vi "Calibration_AH2700.vi"(4 "B-Feld":dbl=4.0, 5 "error in (no error)":errorcluster) -> (15 "Ausgabe-Cluster":T1={" I (A)"=-6.000000000000021, "Voltage"=0.143902, "B-Feld"=4.0, "Timestamp"=3443775799.1979947} {"Timestamp" format="%#_6f"}, 19 "error out":errorcluster)   [LabVIEW 2019]
uses:
  Instrument_Setup.vi
  Global/Global Variables/global.vi
  Instance           2 16Saved   Yokogawa .vi
  Global/Global Variables/Data_Display_global.vi
  <vilib>/Utility/file.llb/Write To Spreadsheet File (DBL).vi
panel:
  out "XY Graph":cluster{dbl[], dbl[]}(graph)={[-6.000000000000005, -4.990000000000027, -3.9901000000000244, -2.9900990000000083, -1.9999999999999865, -0.9900000000000079, 2.400857290751901e-15, 1.000000000000001, 2.0000000000000018, 3.0099999999999802, 4.009899999999982, 5.009900999999998, 6.00000000000002, 4.990000000000042, 3.9901000000000395, 2.999999999999979, 1.9900000000000007, 0.9999999999999987, -1.5439038936193583e-15, -1.0000000000000018, -2.0000000000000027, -3.009999999999981, -4.009899999999983, -5.009900999999999, -6.000000000000021], [0.1439003448275862, 0.14384071428571427, 0.14379167857142858, 0.14374593103448274, 0.14371203448275863, 0.14368321428571423, 0.1436658620689656, 0.1436561034482759, 0.14365485714285722, 0.14366034482758627, 0.14367178571428574, 0.1436978571428571, 0.14372814285714283, 0.14369535714285714, 0.1436752857142857, 0.14366071428571434, 0.14365396428571436, 0.14365448275862072, 0.14366448275862076, 0.14368586206896547, 0.1437107142857143, 0.14374785714285715, 0.14379375862068966, 0.1438423214285714, 0.1439047142857143]}
  in  "file path (dialog if empty)":path=path "D:/UserData/Matthias/Messungen/MgOZnO/130215/130215_259a_kalib4T_1.txt"
  out "Done":bool=TRUE
  out "Data":bool
  out "UI":dbl=-6.000000000000021
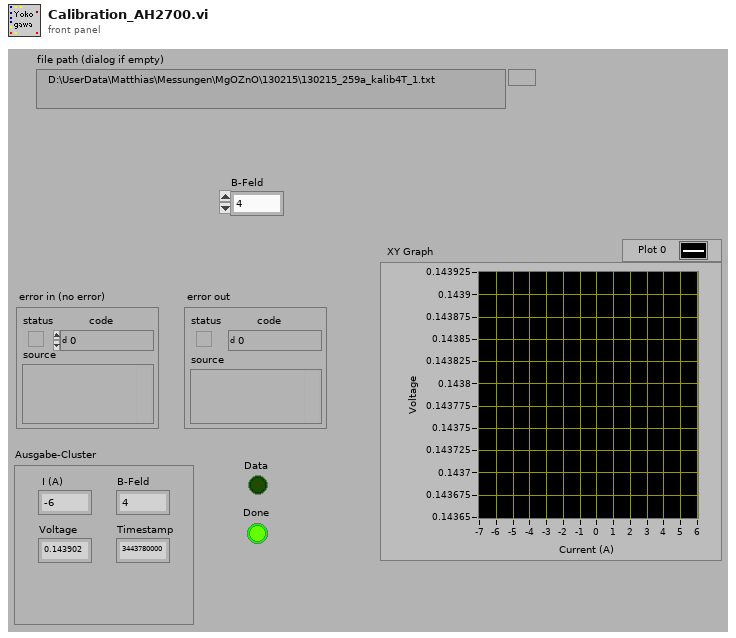
[diagram p1: front panel]
types:
  T1 = cluster{" I (A)":dbl, "Voltage":dbl, "B-Feld":dbl, "Timestamp":dbl}
  T2 = cluster{"UI":dbl, "Capacity":dbl, "B-Feld":dbl, dbl}
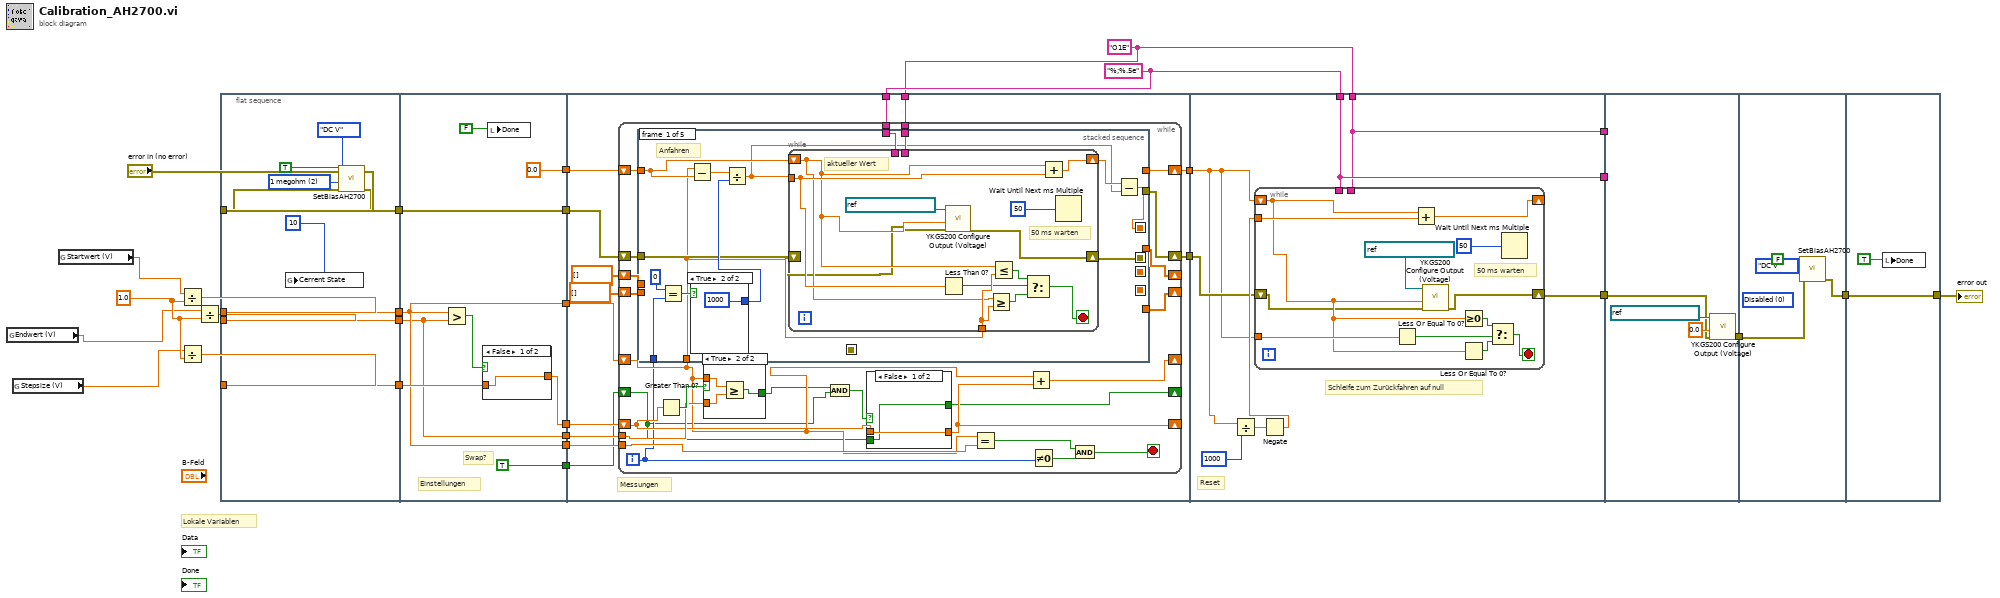
[diagram p0: block diagram]
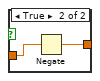
[diagram p2: hidden frame]
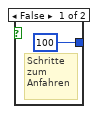
[diagram p3: hidden frame]
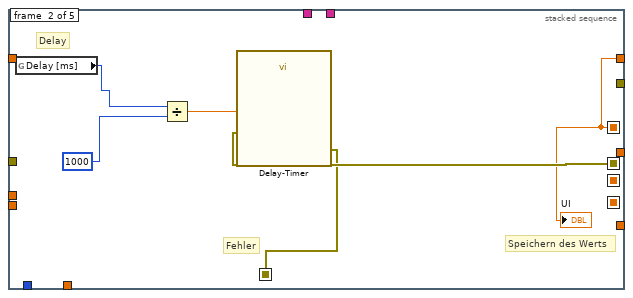
[diagram p4: hidden frame]
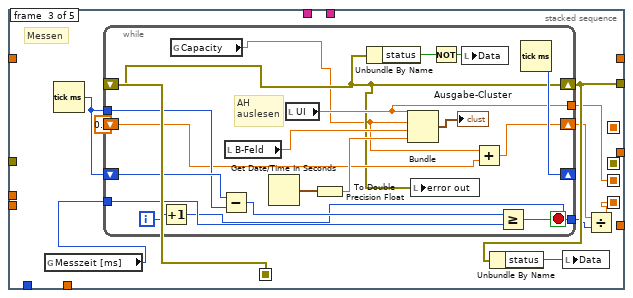
[diagram p5: hidden frame]
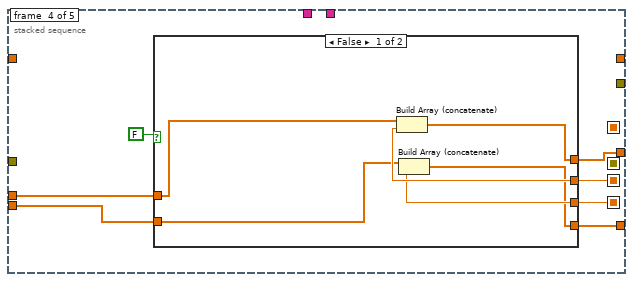
[diagram p6: hidden frame]
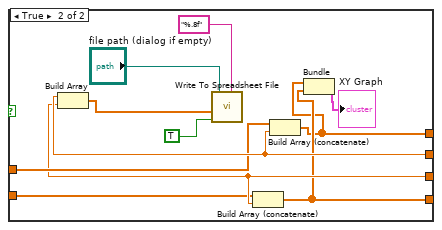
[diagram p7: hidden frame]
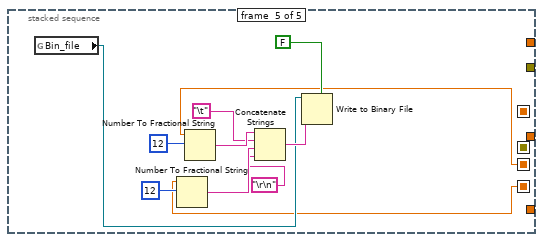
[diagram p8: hidden frame]
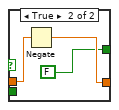
[diagram p9: hidden frame]
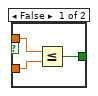
[diagram p10: hidden frame]
diagram:
  w10 = 1.0 ("y")
  w19 = "O1E"
  w20 = "%;%.5e"
  # "Lokale Variablen"
  n1 = global read "Instrument_Setup.vi" "Endwert (V)"() -> (w2:dbl)
  n2 = global read "Instrument_Setup.vi" "Stepsize (V)"() -> (w1:dbl)
  n3 = global read "Instrument_Setup.vi" "Startwert (V)"() -> (w3:dbl)
  n4 = Divide(x=w3, y=w10) -> (x/y=w13:dbl)
  n5 = Divide(x=w1, y=w10) -> (x/y=w11:dbl)
  n6 = Divide(x=w2, y=w10) -> (x/y=w12:dbl)
  n7 = flat-sequence {
    tunnel: "error in (no error)" -> [w34]
    tunnel: w11 -> [w36]
    tunnel: w12 -> [w37]
    tunnel: w13 -> [w38]
    tunnel: [w38] -> w9
    tunnel: [w37] -> w8
    tunnel: [w36] -> w7
    tunnel: [w33] -> w6
    tunnel: [w44] -> w29
    tunnel: [w45] -> w28
    tunnel: [w44] -> w27
    tunnel: [w43] -> w26
    tunnel: [0.0] -> w25
    tunnel: [w39] -> w24
    tunnel: [TRUE] -> w23
    tunnel: w9 -> [w44]
    tunnel: w8 -> [w43]
    tunnel: w7 -> [w46]
    tunnel: w6 -> [w39]
    tunnel: w29 -> [w63]
    tunnel: w28 -> [w61]
    tunnel: w27 -> [w62]
    tunnel: w26 -> [w60]
    tunnel: w25 -> [w59]
    tunnel: w20 -> [w58]
    tunnel: w19 -> [w57]
    tunnel: w24 -> [w56]
    tunnel: w23 -> [w54]
    tunnel: [w55] -> w22
    tunnel: [w53] -> w21
    tunnel: w22 -> [w202]
    tunnel: w21 -> [w200]
    tunnel: w20 -> [w199]
    tunnel: w19 -> [w198]
    tunnel: [w201] -> w17
    tunnel: [w199] -> w15
    tunnel: [w198] -> w14
    tunnel: w17 -> [w219]
    tunnel: w15 -> [_]
    tunnel: w14 -> [_]
    tunnel: [w218] -> w4
    tunnel: [w225] -> w5
    tunnel: w4 -> [w222]
    tunnel: [w227] -> w18
    tunnel: w5 -> [w227]
    frame #0 {
      w31 = 2 items=["Disabled", "100 megohm", "1 megohm"] ("Bias (Off)")
      n8 = global write "global.vi" "Cerrent State"(10) -> ()
      n9 = call "SetBiasAH2700.vi"("error in (no error)"=w34, "Bias (Off)"=w31, "V/A ?"=enum16{"DC V", "DC A"}."DC V", "On/Off"=TRUE) -> ("error out"=w33:errorcluster)  [unwired: 7 in]
    }
    frame #1 {
      # "Einstellungen"
      # "Swap?"
      n10 = Greater?(x=w44, y=w43) -> (0:w47:bool)
      n11 = case shown="False" w47 {
        tunnel: w46 -> [w48 w50]
        tunnel: [w48 w49] -> w45
        frame False {
        }
        frame True {
          n12 = Negate(x=w50) -> (-x=w49:dbl)
        }
      }
      n13 = local write "Done"(FALSE) -> ()
    }
    frame #2 {
      # "Messungen"
      n14 = while {
        shift-right: [w77] -> _
        shift-left: w63 -> [w79]
        tunnel: w62 -> [w88]
        shift-right: [w78] -> _
        shift-left: w61 -> [w85]
        tunnel: w60 -> [w86]
        shift-right: [w80] -> w53
        shift-left: w59 -> [w84]
        tunnel: w58 -> [w83]
        tunnel: w57 -> [w82]
        shift-right: [w76] -> w55
        shift-left: w56 -> [w81]
        shift-right: [w71] -> _
        shift-left: w54 -> [w69]
        shift-right: [w66] -> _
        shift-left: dbl[] [] -> [w67]
        shift-right: [w65] -> _
        shift-left: dbl[] [] -> [w64]
        i -> [w75]
        stop <- w72 stop-if-true
        n15 = stacked-sequence {
          seq-local: [w94 _ _ _ _] -> [_ w122 _ _ _]
          seq-local: [_ w121 _ _ _] -> [_ _ w131 _ _]
          seq-local: [w89 _ _ _ _] -> [_ w118 _ _ _]
          seq-local: [_ _ w127 _ _] -> [_ _ _ w158 w177]
          seq-local: [_ _ w124 _ _] -> [_ _ _ w156 w176]
          tunnel: w75 -> [w101 _ _ _ _]
          tunnel: w84 -> [w93 _ _ _ _]
          tunnel: w79 -> [w92 _ _ _ _]
          tunnel: w83 -> [w97 _ _ _ _]
          tunnel: w82 -> [w96 _ _ _ _]
          tunnel: w81 -> [w95 _ _ _ _]
          tunnel: [_ w118 _ _ _] -> w80
          tunnel: [_ _ w130 _ _] -> w76
          tunnel: w67 -> [_ _ _ w157 _]
          tunnel: [_ _ _ w153 _] -> w66
          tunnel: [_ _ _ w154 _] -> w65
          tunnel: w64 -> [_ _ _ w155 _]
          frame #0 {
            # "Anfahren"
            n16 = Equal?(x=0, y=w101) -> (x = y?=w102:bool)
            n17 = Subtract(x=w92, y=w93) -> (x-y=w99:dbl)
            n18 = case shown="True" w102 {
              tunnel: [100 1000] -> w98
              frame False {
                # "Schritte\nzum\nAnfahren"
              }
              frame True {
              }
            }
            n19 = Divide(x=w99, y=w98) -> (x/y=w90:dbl)
            n20 = while {
              shift-right: [w114] -> w91
              shift-left: w93 -> [w106]
              tunnel: w92 -> [w111]
              tunnel: w90 -> [w112]
              tunnel: w97 -> [_]
              tunnel: w96 -> [_]
              shift-right: [w103] -> w94
              shift-left: w95 -> [w105]
              stop <- w107 stop-if-true
              # "50 ms warten"
              # "aktueller Wert"
              n21 = Less Than 0?(x=w112) -> (x < 0?=w110:bool)
              n22 = call "YKGS200 Configure Output (Voltage).vi"("error in (no error)"=w105, "Voltage Level (0.0 V)"=w106, "VISA resource name"=refnum<visa-resource-name> "GPIB0::6::INSTR") -> ("error out"=w103:errorcluster)  [unwired: 7 in, 1 out]
              n23 = Greater Or Equal?(x=w106, y=w111) -> (x >= y?=w108:bool)
              n24 = Less Or Equal?(x=w106, y=w111) -> (x <= y?=w109:bool)
              n25 = Select(t=w109, s=w110, f=w108) -> (s? t:f=w107:bool)
              n26 = Add(x=w106, y=w112) -> (x+y=w114:dbl)
              n27 = Wait Until Next ms Multiple(millisecond multiple=50) -> ()  [unwired: 1 out]
            }
            n28 = Subtract(x=w91, y=w90) -> (x-y=w89:dbl)
          }
          frame #1 {
            # "Delay"
            # "Speichern des Werts"
            # "Fehler"
            n29 = global read "Instrument_Setup.vi" "Delay [ms]"() -> (w117:u32)
            n30 = Divide(x=w117, y=u32 1000) -> (x/y=w119:dbl)
            n31 = call "Delay-Timer"("error in (no error)"=w122, "Delay Time (s)"=w119) -> ("error out"=w121:errorcluster)  [unwired: 9 in]
            "UI" <- w118
          }
          frame #2 {
            # "Messen"
            n32 = global read "Instrument_Setup.vi" "Messzeit [ms]"() -> (w123:u32)
            n33 = Tick Count (ms)() -> (millisecond timer value=w132:u32)
            n34 = while {
              shift-right: [w151] -> _
              shift-left: w132 -> [w150]
              tunnel: w132 -> [w149]
              tunnel: w123 -> [w147]
              shift-right: [w134] -> w130
              shift-left: w131 -> [w134]
              shift-right: [w139] -> w126
              shift-left: 0.0 -> [w138]
              tunnel: [w137] -> w127
              tunnel: [w135] -> w125
              i -> [w136]
              stop <- w148 stop-if-true
              # "AH\nauslesen"
              n35 = Increment(x=w136) -> (x+1=w135:i32)
              n36 = global read "Data_Display_global.vi" "Capacity"() -> (w133:dbl)
              n37 = Subtract(x=w150, y=w149) -> (x-y=w146:u32)
              n38 = local read "B-Feld"() -> (w144:dbl)
              n39 = Get Date/Time In Seconds() -> (seconds since 1Jan1904=w145:timestamp)
              n40 = local read "UI"() -> (w137:dbl)
              n41 = To Double Precision Float(number=w145) -> (double precision float=w143:dbl)
              n42 = Unbundle By Name(w134) -> ("status"=w142:bool)
              n43 = Bundle("UI"=w137, "Capacity"=w133, "B-Feld"=w144, w143) -> (→"Ausgabe-Cluster":T2)  [unwired: 1 in]
              n44 = local write "error out"(w134) -> ()
              n45 = Not(x=w142) -> (.not. x?=w141:bool)
              n46 = local write "Data"(w141) -> ()
              n47 = Add(x=w133, y=w138) -> (x+y=w139:dbl)
              n48 = Greater Or Equal?(x=w146, y=w147) -> (x >= y?=w148:bool)
              n49 = Tick Count (ms)() -> (millisecond timer value=w151:u32)
            }
            n50 = Unbundle By Name(w130) -> ("status"=w129:bool)
            n51 = local write "Data"(w129) -> ()
            n52 = Divide(x=w126, y=w125) -> (x/y=w124:dbl)
          }
          frame #3 {
            n53 = case shown="False" FALSE {
              tunnel: w158 -> [w164 w171]
              tunnel: w157 -> [w160 w170]
              tunnel: w156 -> [w163 w169]
              tunnel: w155 -> [w159 w168]
              tunnel: [w162 w167] -> w154
              tunnel: [w161 w166] -> w153
              frame False {
                n54 = Build Array (concatenate)(w160, w164) -> (w161:dbl[])
                n55 = Build Array (concatenate)(w159, w163) -> (w162:dbl[])
              }
              frame True {
                n56 = Build Array(w171, w169) -> (w175:dbl[])
                n57 = call-poly <vilib>:"Write To Spreadsheet File.vi"("format (%.3f)"="%.8f", "append to file? (new file:F)"=TRUE, "1D data"=w175, "file path (dialog if empty)"="file path (dialog if empty)") -> ()  [unwired: 4 in, 1 out]
                n58 = Build Array (concatenate)(w168, w169) -> (w167:dbl[])
                n59 = Build Array (concatenate)(w170, w171) -> (w166:dbl[])
                n60 = Bundle(w166, w167) -> (→"XY Graph":cluster{dbl[], dbl[]})  [unwired: 1 in]
              }
            }
          }
          frame #4 {
            n61 = global read "Instrument_Setup.vi" "Bin_file"() -> (w182:refnum<file>)
            n62 = Number To Fractional String(number=w176, precision (6)=i16 12) -> (F-format string=w180:string)  [unwired: 2 in]
            n63 = Number To Fractional String(number=w177, precision (6)=i16 12) -> (F-format string=w185:string)  [unwired: 2 in]
            n64 = Concatenate Strings(w185, "\t", w180, "\r\n") -> (w186:string)
            n65 = Write to Binary File ("Write File")(file (use dialog)=w182, data=w186, 5:FALSE ("prepend array or string size? (T)")) -> ()  [unwired: 3 in, 3 out]
          }
        }
        n66 = Greater Than 0?(x=w85) -> (x > 0?=w87:bool)
        n67 = case shown="True" w87 {
          tunnel: w86 -> [w193 w196]
          tunnel: w79 -> [w194 w197]
          tunnel: [w192 w195] -> w70
          frame False {
            n68 = Less Or Equal?(x=w194, y=w193) -> (x <= y?=w192:bool)
          }
          frame True {
            n69 = Greater Or Equal?(x=w197, y=w196) -> (x >= y?=w195:bool)
          }
        }
        n70 = And(x=w70, y=w69) -> (x .and. y?=w68:bool)
        n71 = case shown="False" w68 {
          tunnel: w85 -> [w188 w191]
          tunnel: [w188 w190] -> w78
          tunnel: [w187 FALSE] -> w71
          tunnel: w69 -> [w187 _]
          frame False {
          }
          frame True {
            n72 = Negate(x=w191) -> (-x=w190:dbl)
          }
        }
        n73 = Equal?(x=w79, y=w88) -> (x = y?=w74:bool)
        n74 = Add(x=w79, y=w78) -> (x+y=w77:dbl)
        n75 = Not Equal To 0?(x=w75) -> (x != 0?=w73:bool)
        n76 = And(x=w74, y=w73) -> (x .and. y?=w72:bool)
      }
    }
    frame #3 {
      # "Schleife zum Zurückfahren auf null"
      # "Reset"
      n77 = Divide(x=w200, y=1000) -> (x/y=w204:dbl)
      n78 = Negate(x=w204) -> (-x=w203:dbl)
      n79 = while {
        shift-right: [w212] -> _
        shift-left: w200 -> [w208]
        tunnel: w203 -> [w216]
        tunnel: w199 -> [_]
        tunnel: w198 -> [_]
        shift-right: [w206] -> w201
        shift-left: w202 -> [w207]
        tunnel: w200 -> [w211]
        stop <- w210 stop-if-true
        # "50 ms warten"
        n80 = Less Or Equal To 0?(x=w211) -> (x <= 0?=w215:bool)
        n81 = Add(x=w208, y=w216) -> (x+y=w212:dbl)
        n82 = call "YKGS200 Configure Output (Voltage).vi"("error in (no error)"=w207, "Voltage Level (0.0 V)"=w208, "VISA resource name"=refnum<visa-resource-name> "GPIB0::6::INSTR") -> ("error out"=w206:errorcluster)  [unwired: 7 in, 1 out]
        n83 = Greater Or Equal To 0?(x=w208) -> (x >= 0?=w214:bool)
        n84 = Less Or Equal To 0?(x=w208) -> (x <= 0?=w213:bool)
        n85 = Select(t=w214, s=w215, f=w213) -> (s? t:f=w210:bool)
        n86 = Wait Until Next ms Multiple(millisecond multiple=50) -> ()  [unwired: 1 out]
      }
    }
    frame #4 {
      n87 = call "YKGS200 Configure Output (Voltage).vi"("error in (no error)"=w219, "Voltage Level (0.0 V)"=0.0, "VISA resource name"=refnum<visa-resource-name> "GPIB0::6::INSTR") -> ("error out"=w218:errorcluster)  [unwired: 7 in, 1 out]
    }
    frame #5 {
      (unwired) 0 items=["Disabled", "100 megohm", "1 megohm"] ("Bias (Off)")
      n88 = call "SetBiasAH2700.vi"("error in (no error)"=w222, "V/A ?"=enum16{"DC V", "DC A"}."DC V", "On/Off"=FALSE) -> ("error out"=w225:errorcluster)  [unwired: 8 in]
    }
    frame #6 {
      n89 = local write "Done"(TRUE) -> ()
    }
  }
  "error out" <- w18
